vi "Convert Device Units to Position Units (Polymorphic).vi"   [LabVIEW 2021, in "Zaber A Series.lvlib"]
doc: "Helper to convert device-specific position units to standard units of measure.\n\nPass in a position measurement from a device and a unit to convert to. The output will be the measurement converted to the selected units.\n\nIf you select a unit other than microsteps, you must also provide the Microstep Size conversion factor from microsteps to micrometers (for linear devices) or degrees (for rotary devices), which can be found in your device manual."
uses:
  Zaber A Series.lvlib
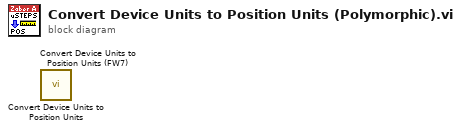
[diagram p0: block diagram]
diagram:
  n1 = call "Convert Device Units to Position Units.vi"() -> ()  [unwired: 11 in, 1 out]
  n2 = call "Convert Device Units to Position Units (FW7).vi"() -> ()  [unwired: 11 in, 1 out]
